vi "Load_Max_Velocity.vi"() -> ()   [LabVIEW 2018]
panel:
  out "Serial Out":refnum<visa-resource-name>
  out "Error Out":errorcluster
  in  "Error In":errorcluster
  in  "Serial In":refnum<visa-resource-name>
  in  "Max. Velocity":i64
  in  "Node":i32
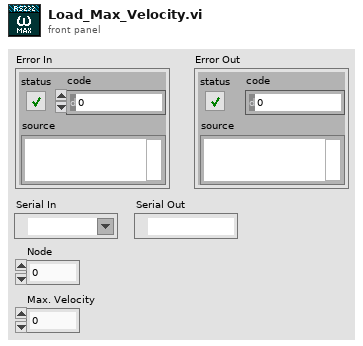
[diagram p1: front panel]
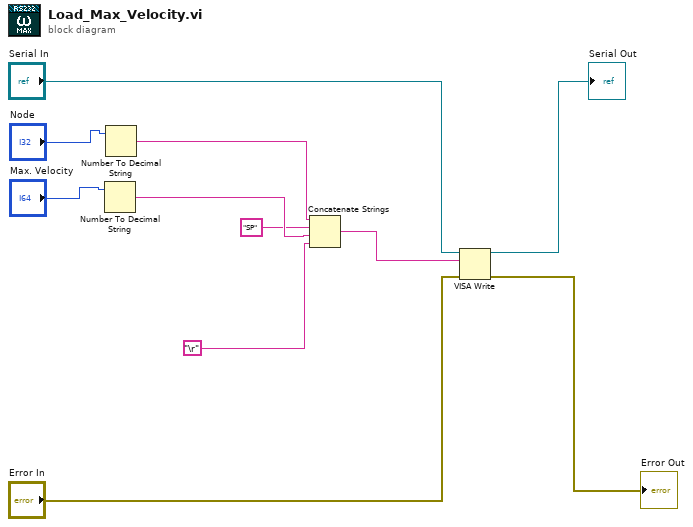
[diagram p0: block diagram]
diagram:
  n1 = Number To Decimal String(number="Max. Velocity") -> (decimal integer string=w3:string)  [unwired: 1 in]
  n2 = Number To Decimal String(number="Node") -> (decimal integer string=w4:string)  [unwired: 1 in]
  n3 = Concatenate Strings(w4, "SP" ("string"), w3, "\r") -> (w2:string)
  n4 = VISA Write(VISA resource name="Serial In", write buffer=w2, error in (no error)="Error In") -> (VISA resource name out=→"Serial Out":refnum<visa-resource-name>, error out=→"Error Out":errorcluster)  [unwired: 1 out]
